vi "Target-Scoped FIFO (2xI16) - Create Resource.vi"() -> (4 "Target-Scoped FIFO (2xI16)":T1)   [LabVIEW 2018, in "Streaming FPGA.lvlib"]
doc: "Creates a Target-scoped FIFO with the data type provided by the <B>Data Type (2xI16).ctl</B>."
uses:
  Streaming FPGA.lvlib
  Target-Scoped FIFO (2xI16) Resource.ctl
  <vilib>/rvi/DataTransferAndStorage/Container/Common/niFpgaContainerGetUniqueNameForEmu.vi
  <vilib>/rvi/DataTransferAndStorage/Container/Common/niFpgaContainerSetEmuInfo.vi
  <vilib>/rvi/eio/common/nirviEmuReportErrorAndStop.vi
  <vilib>/rvi/LocalResourceManager/LocalResourceManager.xnode
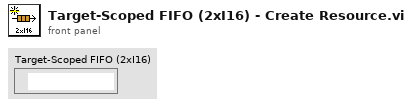
[diagram p1: front panel]
types:
  T1 = typedef "Streaming FPGA.lvlib/Target-Scoped FIFO (2xI16) Resource.ctl" = refnum<k21>
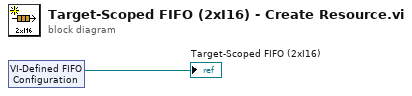
[diagram p0: block diagram]
diagram:
  n1 = xnode "VI-Defined FIFO Configuration"() -> ("FIFO Out"=→"Target-Scoped FIFO (2xI16)":refnum<k21>)
